vi "SVXMPL_Measurement Settled.vi"(0 "value in":dbl format="%.2f", 1 "settling type":enum16{"Linear", "Exponential"}(ring), 2 "settling [iterations]":i32=1 min=1, 5 "tolerance":dbl=0.1 format="%.2f", 7 "tolerance units":T1(ring), 9 "dB reference or full scale value":dbl=1.0 format="%.2f", 11 "error in":errorcluster, 12 "reset":bool, 13 "timeout [iterations]":i32=100 min=1) -> (4 "dup value":dbl format="%.2f", 10 "settled":bool, 15 "error out":errorcluster)   [LabVIEW 2017]
doc: "This example VI applies the specified settling parameters to the values input to the VI. This VI is expected to be called in a loop.\n\n<B>settling type</B> can be set to \"Linear\" or \"Exponential.\" For \"Linear\" settling, the measurement is settled if the measured values for the last settling [iterations] are such that |(max value) - (min value)| <= 2 * tolerance. For \"Exponential\" settling, the measurement is settled if the following conditions are true:\nvalue(N) - value(N-1) <= tolerance\nvalue(N-1) - value(N-2) <= tolerance *2\nvalue(N-2) - value(N-3) <= tolerance *2^2\n...\nvalue(N-settling [iterations]) - value(N-settling [iterations]-1) <= tolerance *2^settling [iterations]\n\nSet <B>tolerance</B> and <B>tolerance units</B> according to the measurement requirements. If you select \"dB\" or \"% full scale\" in <B>tolerance units</B> set the dB reference or full scale value, respectively in <B>dB reference or full scale value</B>.\n\nSet <B>timeout [iterations]</B> to be the maximum allowable number of iterations this VI can be called to test the measurement against the settling criteria before an error -10800 will be generated."
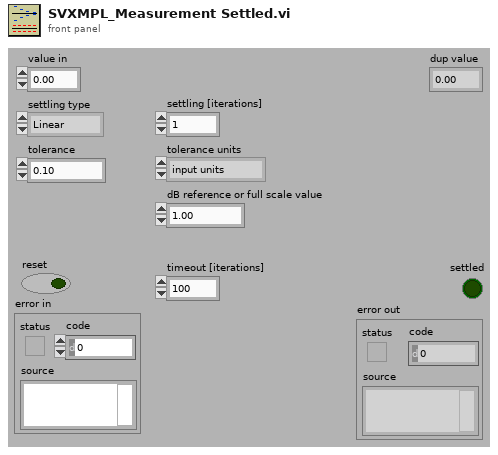
[diagram p1: front panel]
types:
  T1 = enum16{"input units", "% of value", "% of full scale", "dB"}
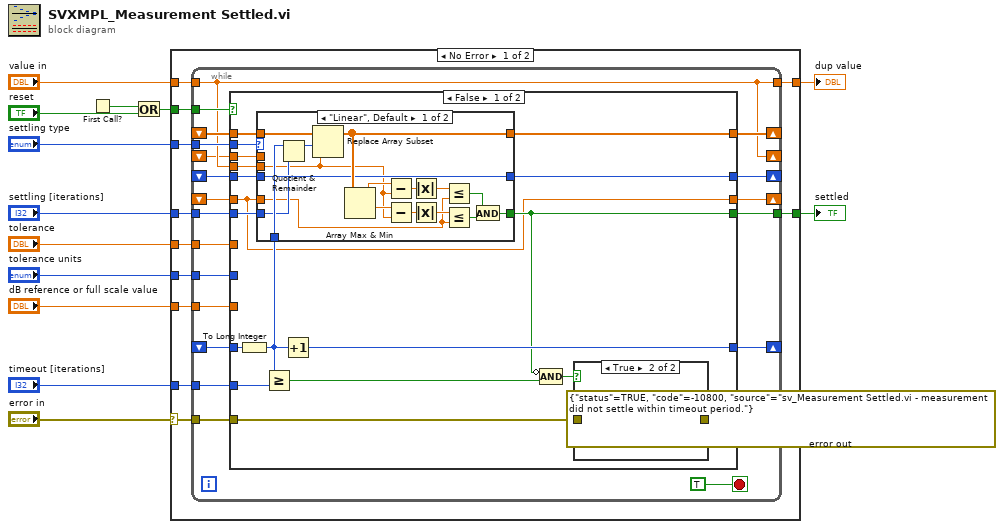
[diagram p0: block diagram]
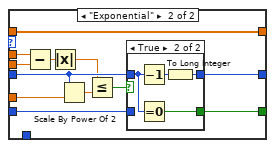
[diagram p2: hidden frame]
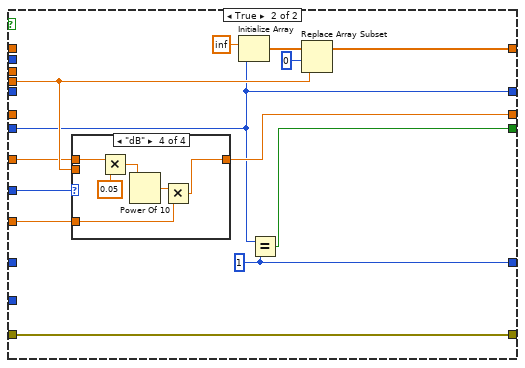
[diagram p5: hidden frame]
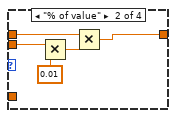
[diagram p7: hidden frame]
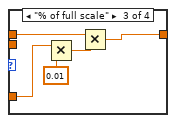
[diagram p8: hidden frame]
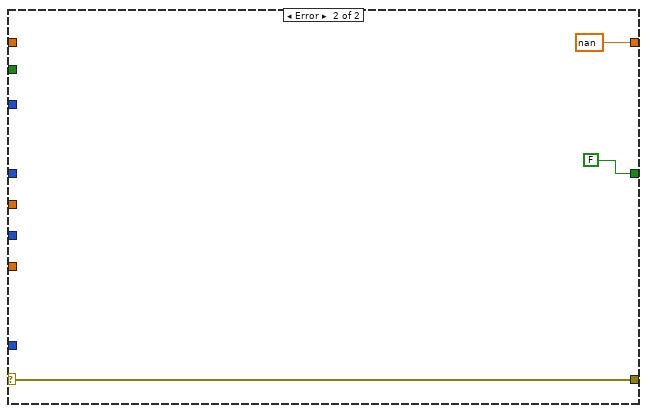
[diagram p9: hidden frame]
diagram:
  n1 = First Call?() -> (First Call?: T/F=w1:bool)
  n2 = Or(x=w1, y="reset") -> (x .or. y?=w7:bool)
  n3 = case shown="No Error" "error in" {
    selector: "error in" -> [w22 w135]
    tunnel: [w19 w135] -> w13
    tunnel: "value in" -> [w26 _]
    tunnel: [w25 nan ("value in")] -> w11
    tunnel: [w20 FALSE ("settled")] -> w10
    tunnel: "settling type" -> [w24 _]
    tunnel: w7 -> [w23 _]
    tunnel: "timeout [iterations]" -> [w21 _]
    tunnel: "tolerance units" -> [w18 _]
    tunnel: "tolerance" -> [w17 _]
    tunnel: "settling [iterations]" -> [w16 _]
    tunnel: "dB reference or full scale value" -> [w15 _]
    frame No Error {
      n4 = while {
        shift-left: _ -> [w27]
        shift-right: [w28] -> _
        shift-left: _ -> [w31]
        shift-right: [w32] -> _
        shift-left: _ -> [w29]
        shift-right: [w30] -> _
        shift-left: _ -> [w33]
        shift-right: [w34] -> _
        tunnel: w15 -> [w35]
        tunnel: w16 -> [w36]
        tunnel: w17 -> [w37]
        tunnel: w18 -> [w38]
        tunnel: [w39] -> w19
        tunnel: [w40] -> w20
        tunnel: w21 -> [w42]
        tunnel: w22 -> [w45]
        tunnel: w23 -> [w46]
        tunnel: w24 -> [w44]
        tunnel: w26 -> [w32]
        tunnel: [w32] -> w25
        shift-left: _ -> [w43]
        shift-right: [w41] -> _
        stop <- TRUE stop-if-true
        n5 = case shown="False" w46 {
          tunnel: w44 -> [w53 _]
          tunnel: w43 -> [w64 _]
          tunnel: w45 -> [w49 w114]
          tunnel: w42 -> [w65 _]
          tunnel: [w63 w113] -> w41
          tunnel: [w54 w115] -> w40
          tunnel: [w62 w114] -> w39
          tunnel: w32 -> [w55 w108]
          tunnel: w38 -> [_ w106]
          tunnel: w37 -> [_ w107]
          tunnel: w36 -> [w58 w103]
          tunnel: w35 -> [_ w105]
          tunnel: [w57 w110] -> w34
          tunnel: w33 -> [w56 _]
          tunnel: w31 -> [w52 _]
          tunnel: [w51 w103] -> w30
          tunnel: w29 -> [w50 _]
          tunnel: [w48 w104] -> w28
          tunnel: w27 -> [w48 _]
          frame False {
            n6 = To Long Integer(number=w64) -> (32bit integer=w59:i32)
            n7 = case shown="\"Linear\", Default" w53 {
              tunnel: w59 -> [w82 _]
              tunnel: w58 -> [w69 w87]
              tunnel: [w80 w84] -> w57
              tunnel: w56 -> [w79 w84]
              tunnel: w55 -> [w68 w89]
              tunnel: w48 -> [w67 w91]
              tunnel: [w75 w86] -> w54
              tunnel: w52 -> [_ w90]
              tunnel: [w70 w88] -> w51
              tunnel: w50 -> [w70 w85]
              frame "Linear", Default {
                n8 = Quotient & Remainder(x=w82, y=w69) -> (x-y*floor(x/y)=w81:i32)  [unwired: 1 out]
                n9 = Replace Array Subset(array=w79, new element=w68, index=w81) -> (w80:dbl[])
                n10 = Array Max & Min(array=w80) -> (max value=w71:dbl, min value=w78:dbl)  [unwired: 2 out]
                n11 = Subtract(x=w71, y=w68) -> (x-y=w77:dbl)
                n12 = Subtract(x=w78, y=w68) -> (x-y=w76:dbl)
                n13 = Absolute Value(x=w77) -> (abs(x)=w74:dbl)
                n14 = Absolute Value(x=w76) -> (abs(x)=w73:dbl)
                n15 = Less Or Equal?(x=w74, y=w67) -> (x <= y?=w66:bool)
                n16 = Less Or Equal?(x=w73, y=w67) -> (x <= y?=w72:bool)
                n17 = And(x=w66, y=w72) -> (x .and. y?=w75:bool)
              }
              frame "Exponential" {
                n18 = Subtract(x=w90, y=w89) -> (x-y=w94:dbl)
                n19 = Absolute Value(x=w94) -> (abs(x)=w83:dbl)
                n20 = Scale By Power Of 2(n=w85, x=w91) -> (x*2^n=w93:dbl)
                n21 = Less Or Equal?(x=w83, y=w93) -> (x <= y?=w92:bool)
                n22 = case shown="True" w92 {
                  selector: w92 -> [w95 _]
                  tunnel: w85 -> [_ w98]
                  tunnel: [w96 w100] -> w88
                  tunnel: [w95 w97] -> w86
                  tunnel: w87 -> [w96 _]
                  frame False {
                  }
                  frame True {
                    n23 = Decrement(x=w98) -> (x-1=w99:i32)
                    n24 = Equal To 0?(x=w98) -> (x = 0?=w97:bool)
                    n25 = To Long Integer(number=w99) -> (32bit integer=w100:i32)
                  }
                }
              }
            }
            n26 = Greater Or Equal?(x=w59, y=w65) -> (x >= y?=w61:bool)
            n27 = Increment(x=w59) -> (x+1=w63:i32)
            n28 = Compound Arithmetic op=AND(invert w54, w61) -> (w60:bool)
            n29 = case shown="True" w60 {
              tunnel: w49 -> [w101 _]
              tunnel: [w101 errorcluster {"status"=TRUE, "code"=-10800, "source"="sv_Measurement Settled.vi - measurement did not settle within timeout period."} ("error IO")] -> w62
              frame False {
              }
              frame True {
              }
            }
          }
          frame True {
            w113 = 1
            n30 = case shown="\"dB\"" w106 {
              tunnel: [w116 w117 w122 w127] -> w104
              tunnel: w107 -> [w116 w121 w125 w132]
              tunnel: w105 -> [_ _ w124 w128]
              tunnel: w108 -> [_ w120 _ _]
              frame "input units", Default {
              }
              frame "% of value" {
                n31 = Multiply(x=w120, y=0.01) -> (x*y=w118:dbl)
                n32 = Multiply(x=w121, y=w118) -> (x*y=w117:dbl)
              }
              frame "% of full scale" {
                n33 = Multiply(x=w124, y=0.01) -> (x*y=w123:dbl)
                n34 = Multiply(x=w125, y=w123) -> (x*y=w122:dbl)
              }
              frame "dB" {
                n35 = Multiply(x=w132, y=0.05) -> (x*y=w130:dbl)
                n36 = Power Of 10(x=w130) -> (10^x=w129:dbl)
                n37 = Multiply(x=w129, y=w128) -> (x*y=w127:dbl)
              }
            }
            n38 = Initialize Array(inf ("Element Data"), w103) -> (w111:dbl[])
            n39 = Equal?(x=w103, y=w113) -> (x = y?=w115:bool)
            n40 = Replace Array Subset(array=w111, new element=w108, index=0 ("Index")) -> (w110:dbl[])
          }
        }
      }
    }
    frame Error {
    }
  }
  "error out" <- w13
  "dup value" <- w11
  "settled" <- w10
